vi "VT100_ESC.vi"(8 "cursor in":i32, 9 "index in":i32, 10 "Original data":u8[](array[numeric]) format="%.0o", 11 "Data in":u8[](array[numeric])) -> (0 "cursor out":i32, 2 "index out":i32, 3 "Data out":u8[](array[numeric]))   [LabVIEW 2022 SP3]
panel:
  out "scroll":i32[](array[numeric])
  out "Console fixed":string
  out "remove":string
  out "Margins":i32[](array[numeric])
  out "string":string
  out "blank":string
  out "params":string
  out "cmd":string
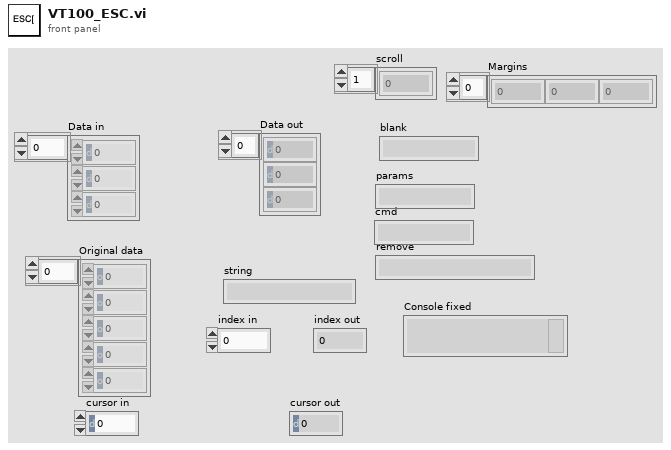
[diagram p1: front panel]
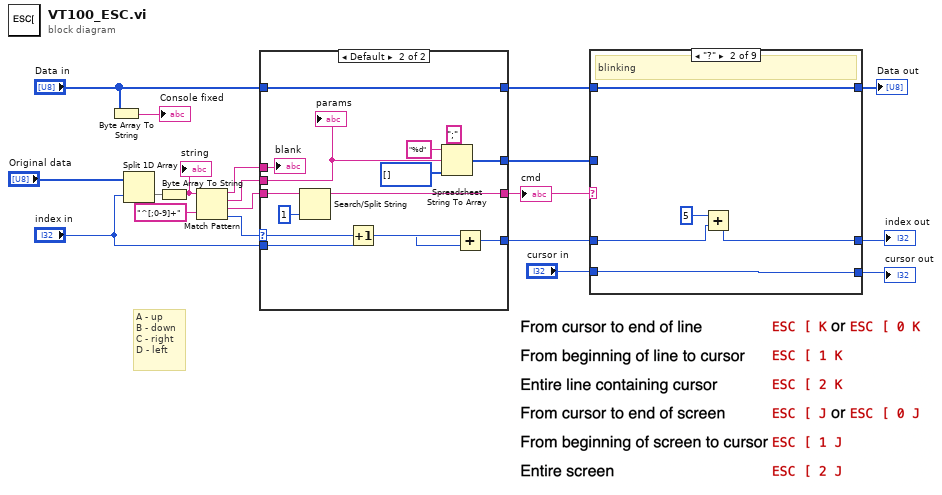
[diagram p0: block diagram]
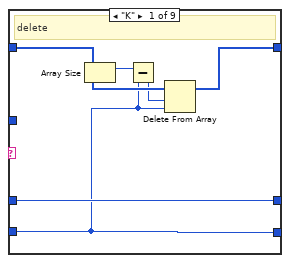
[diagram p2: hidden frame]
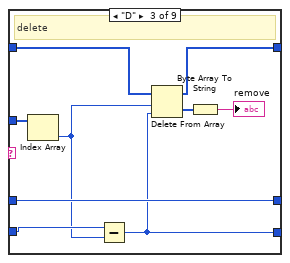
[diagram p3: hidden frame]
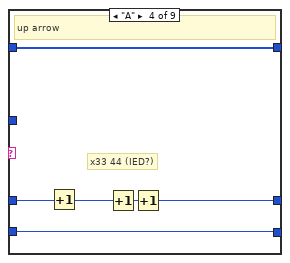
[diagram p4: hidden frame]
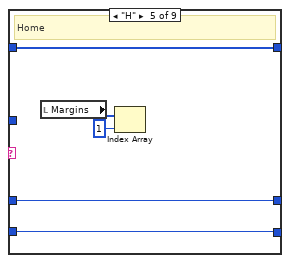
[diagram p5: hidden frame]
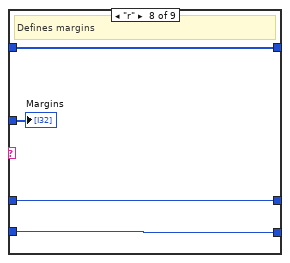
[diagram p8: hidden frame]
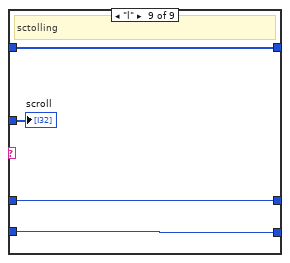
[diagram p9: hidden frame]
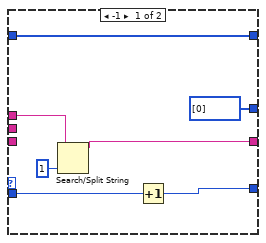
[diagram p10: hidden frame]
diagram:
  # "A - up\nB - down\nC - right\nD - left"
  n1 = Byte Array To String(unsigned byte array="Data in") -> (string=→"Console fixed":string)
  n2 = Split 1D Array(array="Original data", index="index in") -> (second subarray=w17:u8[])  [unwired: 1 out]
  n3 = Byte Array To String(unsigned byte array=w17) -> (string=w18:string)
  "string" <- w18
  n4 = Match Pattern(string=w18, regular expression="^[;0-9]+") -> (before substring=w16:string, match substring=w15:string, after substring=w14:string, offset past match=w13:i32)  [unwired: 1 in]
  n5 = case shown="Default" w13 {
    selector: w13 -> [_ w38]
    tunnel: [w25 w33] -> w10
    tunnel: "Data in" -> [w25 w33]
    tunnel: "index in" -> [w26 w40]
    tunnel: [w21 w39] -> w8
    tunnel: w16 -> [w23 w37]
    tunnel: w15 -> [_ w27]
    tunnel: w14 -> [_ w35]
    tunnel: [w22 w32] -> w12
    tunnel: [i32[] [0] w28] -> w9
    frame -1 {
      n6 = Search/Split String(string=w23, offset (0)=1) -> (substring before match=w22:string)  [unwired: 1 in, 2 out]
      n7 = Increment(x=w26) -> (x+1=w21:i32)
    }
    frame Default {
      n8 = Search/Split String(string=w35, offset (0)=1) -> (substring before match=w32:string)  [unwired: 1 in, 2 out]
      n9 = Increment(x=w38) -> (x+1=w34:i32)
      n10 = Spreadsheet String To Array(delimiter (Tab)=";", format string="%d", spreadsheet string=w27, array type (2D Dbl)=i32[] []) -> (array=w28:i32[])
      n11 = Add(x=w40, y=w34) -> (x+y=w39:i32)
      "params" <- w27
      "blank" <- w37
    }
  }
  "cmd" <- w12
  n12 = case shown="\"?\"" w12 {
    tunnel: [w45 w47 w59 w66 w71 w74 w77 w78 w84] -> w11
    tunnel: w10 -> [w44 w47 w55 w66 w71 w74 w77 w78 w84]
    tunnel: w9 -> [_ _ w60 _ _ _ _ w80 w82]
    tunnel: w8 -> [w46 w50 w58 w63 w69 w73 w76 w81 w85]
    tunnel: [w46 w48 w58 w62 w69 w73 w76 w81 w85] -> w7
    tunnel: "cursor in" -> [w42 w51 w54 w61 w70 w72 w75 w79 w83]
    tunnel: [w42 w51 w52 w61 w70 w72 w75 w79 w83] -> w4
    frame "K" {
      # "delete"
      n13 = Array Size(array=w44) -> (size(s)=w43:i32)
      n14 = Subtract(x=w43, y=w42) -> (x-y=w41:i32)
      n15 = Delete From Array(array=w44, length=w41, index=w42) -> (array with subset deleted=w45:u8[])  [unwired: 1 out]
    }
    frame "?" {
      # "blinking"
      n16 = Add(x=5 ("length"), y=w50) -> (x+y=w48:i32)
    }
    frame "D" {
      # "delete"
      n17 = Index Array(array=w60) -> (element=w53:i32)  [unwired: 1 in]
      n18 = Subtract(x=w54, y=w53) -> (x-y=w52:i32)
      n19 = Delete From Array(array=w55, length=w53, index=w52) -> (deleted portion=w57:u8[], array with subset deleted=w59:u8[])
      n20 = Byte Array To String(unsigned byte array=w57) -> (string=→"remove":string)
    }
    frame "A" {
      # "x33 44 (IED?)"
      # "up arrow"
      n21 = Increment(x=w63) -> (x+1=w64:i32)
      n22 = Increment(x=w64) -> (x+1=w65:i32)
      n23 = Increment(x=w65) -> (x+1=w62:i32)
    }
    frame "H" {
      # "Home"
      n24 = local read "Margins"() -> (w68:i32[])
      n25 = Index Array(array=w68, index=1) -> ()  [unwired: 1 out]
    }
    frame Default {
    }
    frame "m" {
      # "bold and such"
    }
    frame "r" {
      # "Defines margins"
      "Margins" <- w80
    }
    frame "l" {
      # "sctolling"
      "scroll" <- w82
    }
  }
  "Data out" <- w11
  "index out" <- w7
  "cursor out" <- w4
